vi "receiveSerialFeedback.vi"(7 "robotAngles":dbl[](array[numeric])=[45.0, 135.0, 225.0, 315.0] format="%#_13g", 8 "error in (no error)":errorcluster, 9 "Com Serial":T2={"Serial TX"=FALSE, "Porta:"="COM12"}, 10 "Game":refnum<class "Game.lvclass">, 11 "Communication in":refnum<class "Communication.lvclass">) -> (0 "error out":errorcluster, 1 "RobotsFeedback":refnum<class "RobotFeedback.lvclass">[](array[class]), 3 "Communication out":refnum<class "Communication.lvclass">)   [LabVIEW 2021, in "Communication.lvclass"]
uses:
  Communication.lvclass
  Controls/ComSerial.ctl
  Game_class/Game.lvclass
  RobotFeedback/RobotFeedback.lvclass
  Game_class/feedbackStatusInfo.ctl
  Game_class/Game.lvclass/Game.ctl
  RobotFeedback/RobotFeedback.lvclass/RobotFeedback.ctl
  Game_class/Read RobotsFeedback.vi
  RobotFeedback/Read id.vi
  RobotFeedback/Write id.vi
  e0417c2e-124f-4661-ba63-af752af84d35.vi
  RobotFeedback/commCAS.vi
  <vilib>/Instr/_visa.llb/VISA Configure Serial Port (Instr).vi
  <vilib>/Comparison/Less/Less Functor/Less Functor.lvclass
  Utilities_class/Utilities.lvclass
panel:
  in  "feedbackStatusInfo":T1
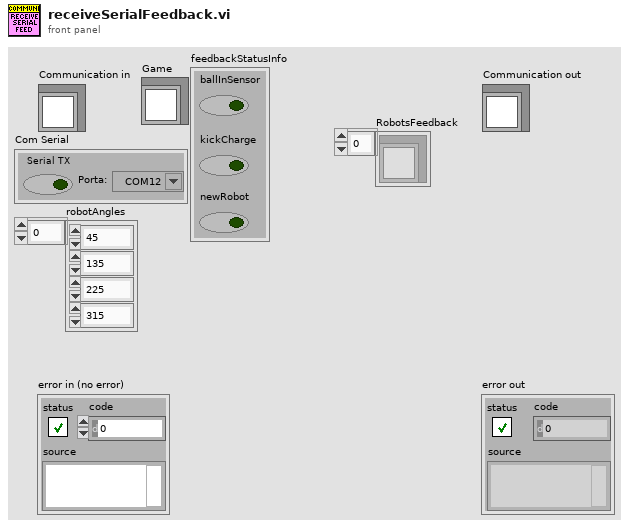
[diagram p1: front panel]
types:
  T1 = typedef "feedbackStatusInfo.ctl" = cluster{"ballInSensor":bool, "kickCharge":bool, "newRobot":bool}
  T2 = typedef "ComSerial.ctl" = cluster{"Serial TX":bool, "Porta:":refnum<visa-resource-name>}
  T3 = typedef "feedbackData.ctl" = cluster{"id":u32, "status":u32, "battery":sgl, "encoder1":sgl, "encoder2":sgl, "encoder3":sgl, "encoder4":sgl}
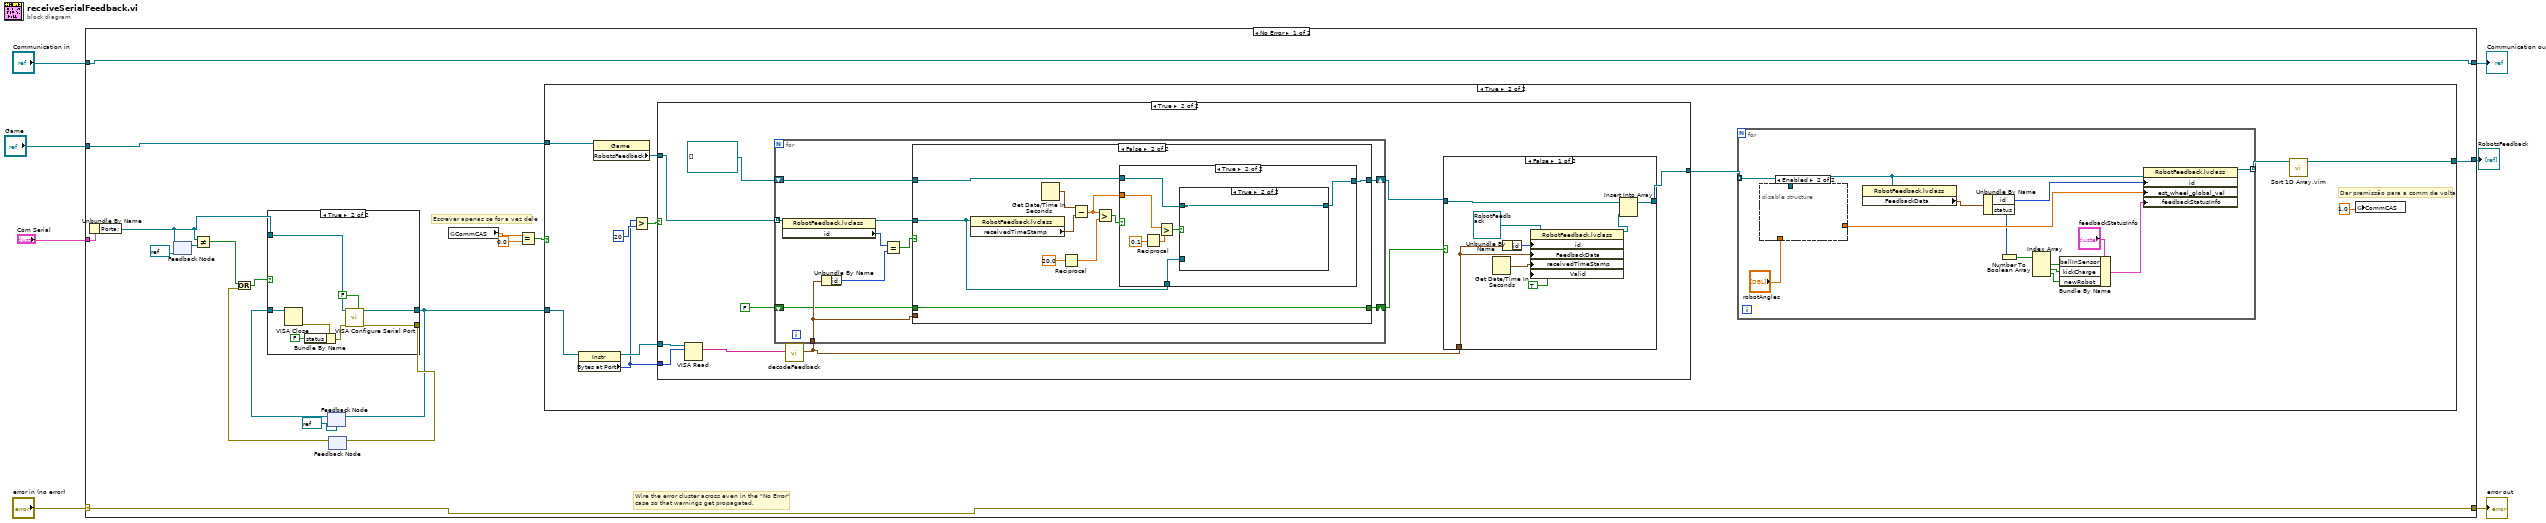
[diagram p0: block diagram]
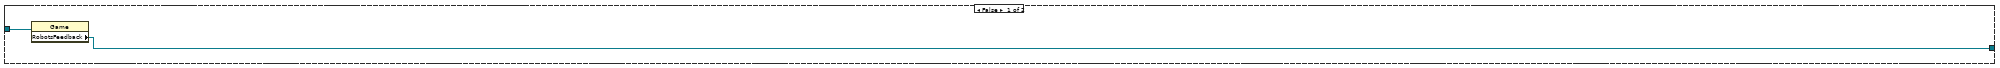
[diagram p2: hidden frame]
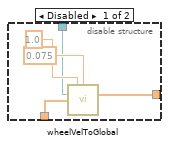
[diagram p3: hidden frame]
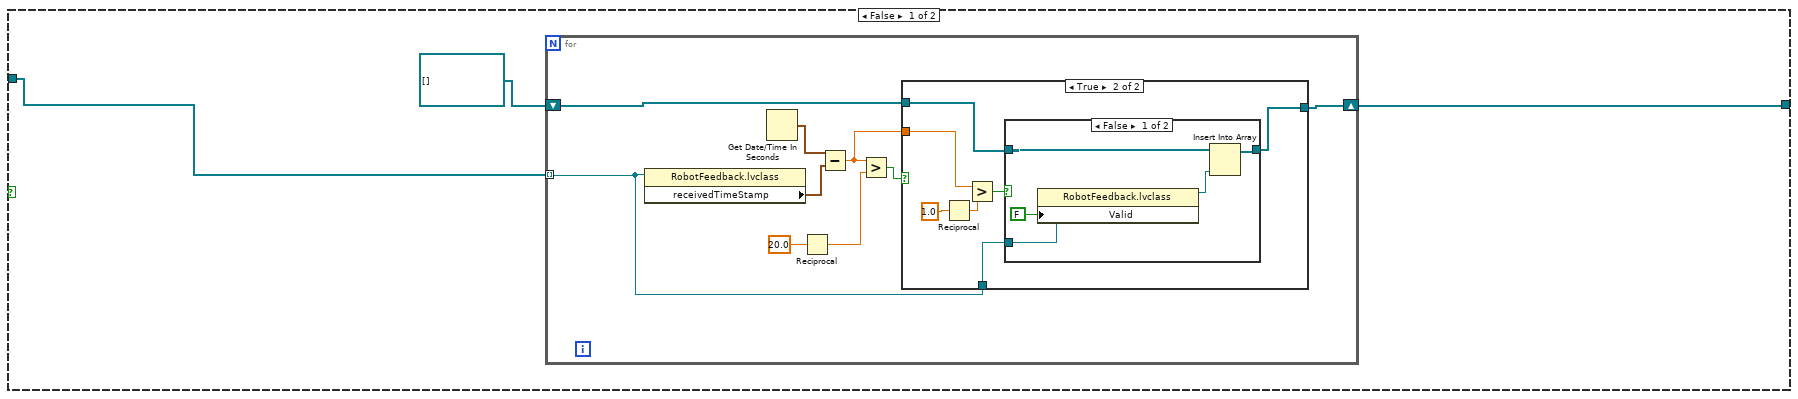
[diagram p4: hidden frame]
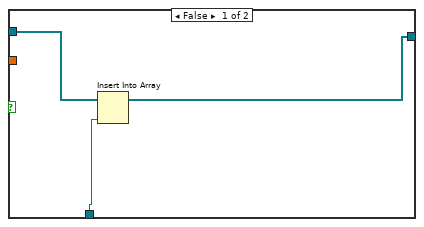
[diagram p5: hidden frame]
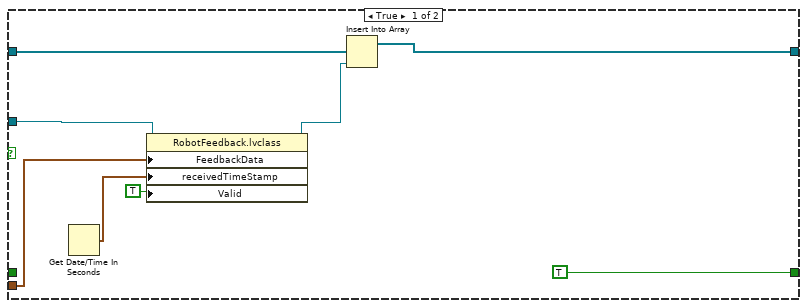
[diagram p8: hidden frame]
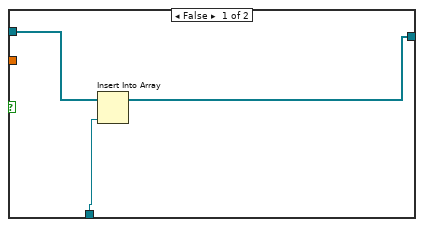
[diagram p9: hidden frame]
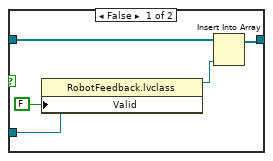
[diagram p10: hidden frame]
diagram:
  n1 = case shown="No Error" "error in (no error)" {
    selector: "error in (no error)" -> [w24 w158]
    tunnel: [w24 w158] -> w6
    tunnel: [w25 w157] -> w4
    tunnel: "Communication in" -> [w25 w157]
    tunnel: "Com Serial" -> [w23 _]
    tunnel: "Game" -> [w13 _]
    tunnel: [w12 _] -> w1
    frame No Error {
      # "Escrever apenas se for a vez dele"
      # "Wire the error cluster across even in the \"No Error\"\ncase so that warnings get propagated."
      n2 = Unbundle By Name(w23) -> ("Porta:"=w14:refnum<visa-resource-name>)
      n3 = feedback #1(refnum<visa-resource-name> refnum ("Porta?")) -> (w22:refnum<visa-resource-name>)
      n4 = feedback-in #1(w14) -> ()
      n5 = Not Equal?(x=w14, y=w22) -> (x != y?=w19:bool)
      n6 = feedback #2(refnum<visa-resource-name> refnum ("VISA resource name out")) -> (w21:refnum<visa-resource-name>)
      n7 = feedback #3() -> (w18:errorcluster)  [unwired: 1 in]
      n8 = Or(x=w19, y=w18) -> (x .or. y?=w15:bool)
      n9 = case shown="True" w15 {
        tunnel: [_ w154] -> w16
        tunnel: [w148 w155] -> w11
        tunnel: w14 -> [_ w150]
        tunnel: w21 -> [w148 w153]
        frame False {
        }
        frame True {
          n10 = VISA Close(VISA resource name=w153) -> (error out=w152:errorcluster)  [unwired: 1 in]
          n11 = Bundle By Name(cluster=w152, "status"=FALSE) -> (w151:errorcluster)
          n12 = call-poly "VISA Configure Serial Port"("VISA resource name"=w150, "Enable Termination\nChar (T)"=FALSE ("Enable Termination\nChar (T)"), "error in (no error)"=w151) -> ("VISA resource name out"=w155:refnum<visa-resource-name>, "error out"=w154:errorcluster)  [unwired: 11 in]
        }
      }
      n13 = feedback-in #2(w11) -> ()
      n14 = feedback-in #3(w16) -> ()
      n15 = global read "commCAS.vi" "CommCAS"() -> (w10:dbl)
      n16 = Equal?(x=w10, y=0.0) -> (x = y?=w8:bool)
      n17 = case shown="True" w8 {
        tunnel: w13 -> [w27 w37]
        tunnel: [w26 w34] -> w12
        tunnel: w11 -> [_ w33]
        frame False {
          n18 = property class="Game"(reference=w27) -> ("RobotsFeedback"=w26:refnum<class "RobotFeedback.lvclass">[])  [unwired: 1 in, 2 out]
        }
        frame True {
          # "Dar premissão para a comm de volta"
          n19 = property class="Instr"(reference=w33) -> (reference out=w32:refnum<visa-resource-name>, "Bytes at Port"=w28:u32)  [unwired: 1 in, 1 out]
          n20 = property class="Game"(reference=w37) -> ("RobotsFeedback"=w38:refnum<class "RobotFeedback.lvclass">[])  [unwired: 1 in, 2 out]
          n21 = Greater?(x=w28, y=u32 20 ("Serial Settings:Number of Bytes at Serial Port")) -> (0:w29:bool)
          n22 = case shown="True" w29 {
            tunnel: w38 -> [w58 w94]
            tunnel: [w57 w90] -> w36
            tunnel: w28 -> [_ w86]
            tunnel: w32 -> [_ w87]
            frame False {
              n23 = for {
                tunnel: w58 -> [w60] mode=indexing
                shift-right: [w67] -> w57
                shift-left: refnum<class "RobotFeedback.lvclass">[] [] -> [w68]
                n24 = property class="RobotFeedback.lvclass"(reference=w60) -> ("receivedTimeStamp"=w65:timestamp)  [unwired: 1 in, 2 out]
                n25 = Get Date/Time In Seconds() -> (seconds since 1Jan1904=w66:timestamp)
                n26 = Reciprocal(x=20.0) -> (1/x=w63:dbl)
                n27 = Subtract(x=w66, y=w65) -> (x-y=w61:dbl)
                n28 = Greater?(x=w61, y=w63) -> (0:w62:bool)
                n29 = case shown="True" w62 {
                  tunnel: w68 -> [w71 w74]
                  tunnel: [w69 w73] -> w67
                  tunnel: w60 -> [w70 w72]
                  tunnel: w61 -> [_ w78]
                  frame False {
                    n30 = Insert Into Array(array=w71, new element=w70) -> (w69:refnum<class "RobotFeedback.lvclass">[])  [unwired: 1 in]
                  }
                  frame True {
                    n31 = Reciprocal(x=1.0) -> (1/x=w76:dbl)
                    n32 = Greater?(x=w78, y=w76) -> (0:w75:bool)
                    n33 = case shown="False" w75 {
                      tunnel: w74 -> [w81 w84]
                      tunnel: [w79 w84] -> w73
                      tunnel: w72 -> [w83 _]
                      frame False {
                        n34 = property class="RobotFeedback.lvclass"(reference=w83, "Valid"=FALSE) -> (reference out=w80:refnum<class "RobotFeedback.lvclass">)  [unwired: 1 in, 1 out]
                        n35 = Insert Into Array(array=w81, new element=w80) -> (w79:refnum<class "RobotFeedback.lvclass">[])  [unwired: 1 in]
                      }
                      frame True {
                      }
                    }
                  }
                }
              }
            }
            frame True {
              n36 = VISA Read(VISA resource name=w87, byte count=w86) -> (read buffer=w85:string)  [unwired: 1 in, 3 out]
              n37 = call "decodeFeedback.vi"("String"=w85) -> ("FeedbackData"=w89:T3)  [unwired: 8 in, 2 out]
              n38 = for {
                tunnel: w94 -> [w111] mode=indexing
                shift-right: [w112] -> w91
                shift-left: refnum<class "RobotFeedback.lvclass">[] [] ("RobotsFeedback") -> [w113]
                tunnel: w89 -> [w107]
                shift-right: [w105] -> w92
                shift-left: FALSE -> [w106]
                n39 = property class="RobotFeedback.lvclass"(reference=w111) -> (reference out=w108:refnum<class "RobotFeedback.lvclass">, "id"=w110:i32)  [unwired: 1 in, 1 out]
                n40 = Unbundle By Name(w107) -> ("id"=w109:u32)
                n41 = Equal?(x=w110, y=w109) -> (x = y?=w104:bool)
                n42 = case shown="False" w104 {
                  tunnel: w113 -> [w121 w127]
                  tunnel: [w116 w126] -> w112
                  tunnel: w108 -> [w120 w125]
                  tunnel: w107 -> [w118 _]
                  tunnel: w106 -> [_ w124]
                  tunnel: [TRUE w124] -> w105
                  frame True {
                    n43 = Get Date/Time In Seconds() -> (seconds since 1Jan1904=w119:timestamp)
                    n44 = property class="RobotFeedback.lvclass"(reference=w120, "FeedbackData"=w118, "receivedTimeStamp"=w119, "Valid"=TRUE) -> (reference out=w117:refnum<class "RobotFeedback.lvclass">)  [unwired: 1 in, 1 out]
                    n45 = Insert Into Array(array=w121, new element=w117) -> (w116:refnum<class "RobotFeedback.lvclass">[])  [unwired: 1 in]
                  }
                  frame False {
                    n46 = property class="RobotFeedback.lvclass"(reference=w125) -> ("receivedTimeStamp"=w130:timestamp)  [unwired: 1 in, 2 out]
                    n47 = Get Date/Time In Seconds() -> (seconds since 1Jan1904=w131:timestamp)
                    n48 = Reciprocal(x=20.0) -> (1/x=w128:dbl)
                    n49 = Subtract(x=w131, y=w130) -> (x-y=w122:dbl)
                    n50 = Greater?(x=w122, y=w128) -> (0:w123:bool)
                    n51 = case shown="True" w123 {
                      tunnel: w127 -> [w134 w137]
                      tunnel: [w132 w136] -> w126
                      tunnel: w125 -> [w133 w135]
                      tunnel: w122 -> [_ w141]
                      frame False {
                        n52 = Insert Into Array(array=w134, new element=w133) -> (w132:refnum<class "RobotFeedback.lvclass">[])  [unwired: 1 in]
                      }
                      frame True {
                        n53 = Reciprocal(x=0.1) -> (1/x=w139:dbl)
                        n54 = Greater?(x=w141, y=w139) -> (0:w138:bool)
                        n55 = case shown="True" w138 {
                          tunnel: w137 -> [w144 w147]
                          tunnel: [w142 w147] -> w136
                          tunnel: w135 -> [w146 _]
                          frame False {
                            n56 = property class="RobotFeedback.lvclass"(reference=w146, "Valid"=FALSE) -> (reference out=w143:refnum<class "RobotFeedback.lvclass">)  [unwired: 1 in, 1 out]
                            n57 = Insert Into Array(array=w144, new element=w143) -> (w142:refnum<class "RobotFeedback.lvclass">[])  [unwired: 1 in]
                          }
                          frame True {
                          }
                        }
                      }
                    }
                  }
                }
              }
              n58 = case shown="False" w92 {
                tunnel: w91 -> [w102 w103]
                tunnel: [w97 w103] -> w90
                tunnel: w89 -> [w99 _]
                frame False {
                  n59 = Get Date/Time In Seconds() -> (seconds since 1Jan1904=w98:timestamp)
                  n60 = Unbundle By Name(w99) -> ("id"=w100:u32)
                  n61 = property class="RobotFeedback.lvclass"(reference=refnum<class "RobotFeedback.lvclass"> refnum ("RobotsFeedback"), "id"=w100, "FeedbackData"=w99, "receivedTimeStamp"=w98, "Valid"=TRUE) -> (reference out=w96:refnum<class "RobotFeedback.lvclass">)  [unwired: 1 in, 1 out]
                  n62 = Insert Into Array(array=w102, new element=w96) -> (w97:refnum<class "RobotFeedback.lvclass">[])  [unwired: 1 in]
                }
                frame True {
                }
              }
            }
          }
          n63 = for {
            tunnel: w36 -> [w49] mode=indexing
            tunnel: [w47] -> w35 mode=indexing
            n64 = disable-structure shown="Enabled" {
              disable-tunnel: "robotAngles" -> [w56 _]
              disable-tunnel: [w53 _] -> w50
              disable-tunnel: w49 -> [w52 _]
              frame Disabled {
                n65 = call "wheelVelToGlobal.vi"("r_wheel"=1.0, "r_robot"=0.075, "RobotsFeedback"=w52, "robotAngles"=w56) -> ("vel_array"=w53:dbl[])  [unwired: 9 in, 2 out]
              }
              frame Enabled {
              }
            }
            n66 = property class="RobotFeedback.lvclass"(reference=w49) -> ("FeedbackData"=w48:T3)  [unwired: 1 in, 2 out]
            n67 = Unbundle By Name(w48) -> ("id"=w46:u32, "status"=w45:u32)
            n68 = Number To Boolean Array(number=w45) -> (Boolean array=w44:bool[])
            n69 = Index Array(array=w44) -> (element #1=w42:bool, element #2=w41:bool, element #3=w40:bool)  [unwired: 3 in]
            n70 = Bundle By Name(cluster="feedbackStatusInfo", "ballInSensor"=w42, "kickCharge"=w41, "newRobot"=w40) -> (w39:T1)
            n71 = property class="RobotFeedback.lvclass"(reference=w49, "id"=w46, "est_wheel_global_vel"=w50, "feedbackStatusInfo"=w39) -> (reference out=w47:refnum<class "RobotFeedback.lvclass">)  [unwired: 1 in, 1 out]
          }
          n72 = call "Sort 1D Array.vim"("unsorted array"=w35) -> ("sorted array"=w34:refnum<class "RobotFeedback.lvclass">[])  [unwired: 10 in]
          n73 = global write "commCAS.vi" "CommCAS"(1.0) -> ()
        }
      }
    }
    frame Error {
    }
  }
  "error out" <- w6
  "Communication out" <- w4
  "RobotsFeedback" <- w1
